vi "Generate Worker Types.vi"(11 "Worker lvlib":path) -> (0 "error out":errorcluster, 1 "Types":T1[](array[typedef]), 2 "Special Terminals":T5={"Action"=-1, "Init"=-1, "Tag"=-1, "State in"=-1, "State out"=-1, "Error"=-1, "Control"=-1}, 3 "Worker VI":refnum<vi>)   [LabVIEW 2022 SP3, in "FlexBlocks Support.lvlib"]
uses:
  FlexBlocks Support.lvlib
  Terminal Direction.ctl
  Value Mode.ctl
  Special Terminal.ctl
  Type Descriptor.ctl
  Special Terminal Indices.ctl
  <vilib>/Utility/Data Type/NI_Data Type.lvlib
  Worker Action.ctl
panel:
  out "Array":path[](array[path])
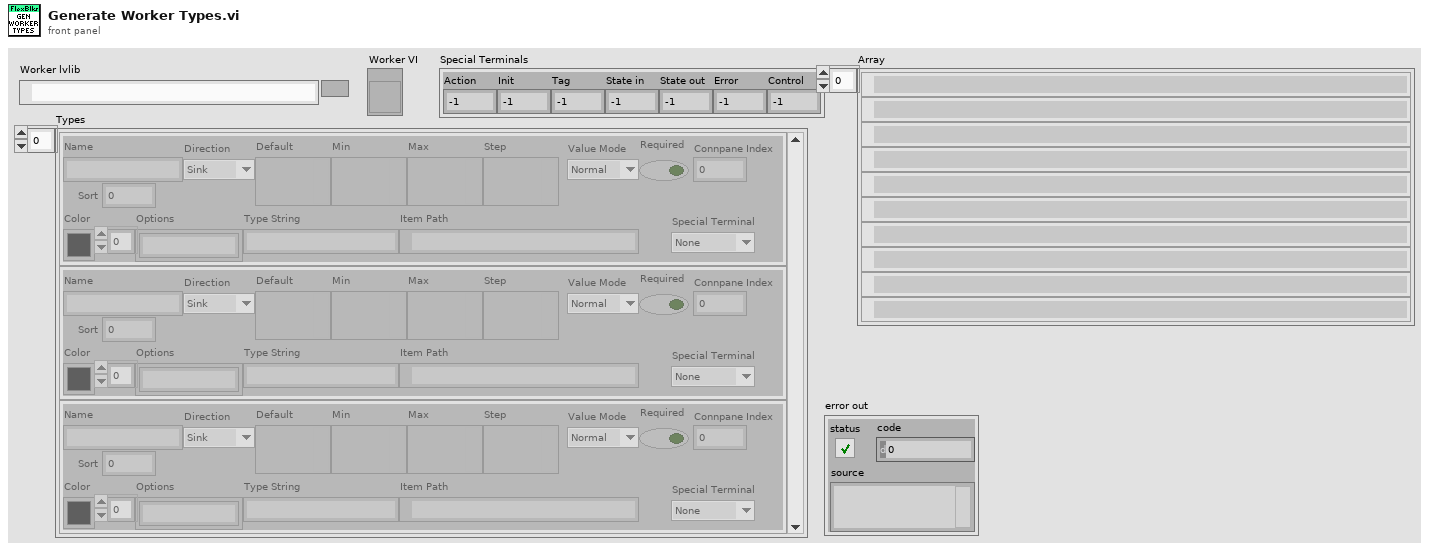
[diagram p1: front panel]
types:
  T1 = typedef "FlexBlocks Support.lvlib/Type Descriptor.ctl" = cluster{"Name":string, "Direction":T2, "Default":variant, "Min":variant, "Max":variant, "Step":variant, "Value Mode":T3, "Color":u32, "Options":string[], "Type String":string, "Item Path":path, "Required":bool, "Connpane Index":i32, "Special Terminal":T4, "Sort":i32}
  T2 = typedef "FlexBlocks Support.lvlib/Terminal Direction.ctl" = enum16{"Sink", "Source"}
  T3 = typedef "FlexBlocks Support.lvlib/Value Mode.ctl" = enum16{"Normal", "Range", "Select"}
  T4 = typedef "FlexBlocks Support.lvlib/Special Terminal.ctl" = enum16{"None", "Action", "Init", "Tag", "State in", "State out", "Error", "Control"}
  T5 = typedef "FlexBlocks Support.lvlib/Special Terminal Indices.ctl" = cluster{"Action":i32, "Init":i32, "Tag":i32, "State in":i32, "State out":i32, "Error":i32, "Control":i32}
  T6 = typedef "FlexBlocks Support.lvlib/Worker Action.ctl" = enum16{"Init", "Start", "Run", "Stop", "Close"}
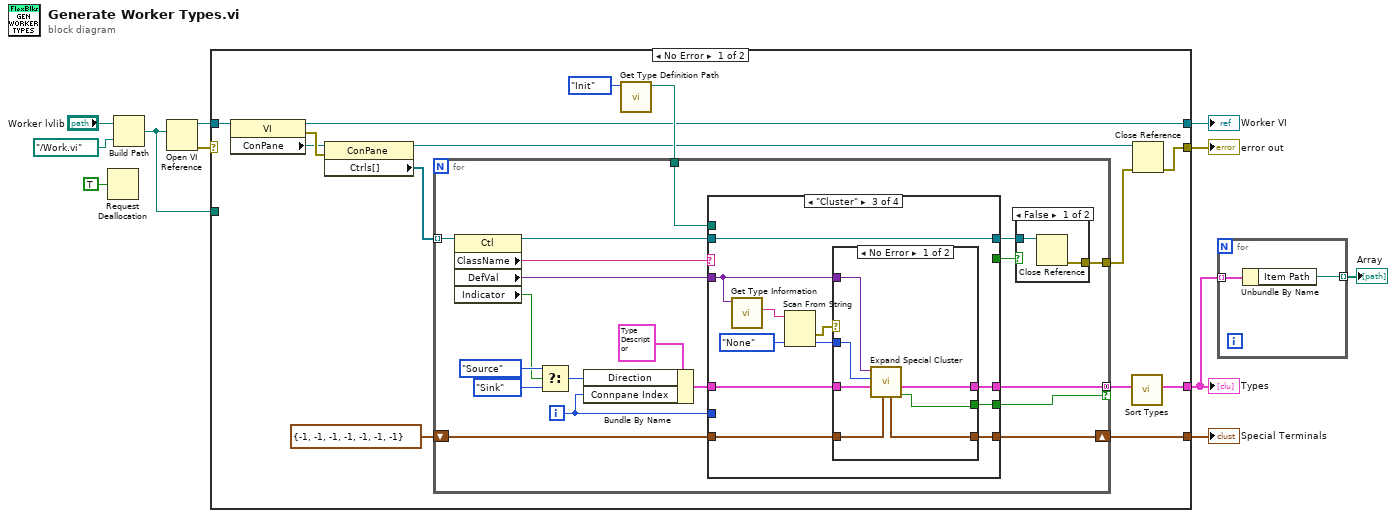
[diagram p0: block diagram]
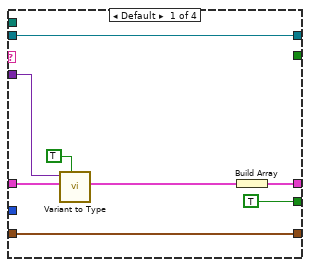
[diagram p3: hidden frame]
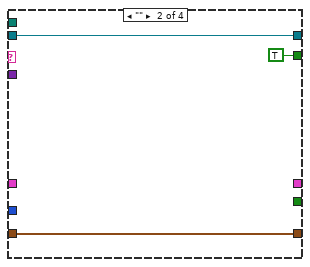
[diagram p4: hidden frame]
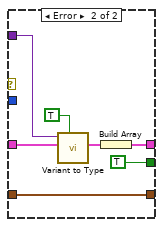
[diagram p5: hidden frame]
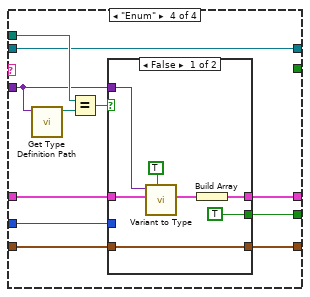
[diagram p6: hidden frame]
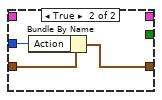
[diagram p7: hidden frame]
diagram:
  n1 = Request Deallocation(TRUE ("flag")) -> ()
  n2 = Build Path(base path="Worker lvlib", name or relative path=path "../Work.vi") -> (appended path=w6:path)
  n3 = Open VI Reference(vi path=w6) -> (vi reference=w8:refnum<vi>, error out=w7:errorcluster)  [unwired: 5 in]
  n4 = case shown="No Error" w7 {
    selector: w7 -> [_ w104]
    tunnel: w8 -> [w23 _]
    tunnel: w6 -> [_ _]
    tunnel: [w14 w104] -> w5
    tunnel: [w18 _] -> w4
    tunnel: [w15 _] -> w3
    tunnel: [w12 _] -> w2
    frame No Error {
      n5 = property class="VI"(reference=w23) -> (reference out=w15:refnum<vi>, error out=w25:errorcluster, "ConPane"=w24:refnum<vi>)  [unwired: 1 in]
      n6 = property class="ConPane"(reference=w24, error in=w25) -> (reference out=w16:refnum<vi>, "Ctrls[]"=w22:refnum<vi>[])  [unwired: 1 out]
      n7 = call <vilib>:"Get Type Definition Path.vi"("variant"=Worker_Action."Init" ("Worker Action")) -> ("type definition path"=w19:path)  [unwired: 9 in, 1 out]
      n8 = for {
        tunnel: w22 -> [w44] mode=indexing
        shift-right: [w32] -> w18
        shift-left: T5 {"Action"=-1, "Init"=-1, "Tag"=-1, "State in"=-1, "State out"=-1, "Error"=-1, "Control"=-1} ("Special Terminal Indices") -> [w38]
        tunnel: w19 -> [w34]
        tunnel: [w30] -> w17
        tunnel: [w29] -> w13 mode=concatenating if=w28
        i -> [w27]
        n9 = property class="Ctl"(reference=w44) -> (reference out=w33:refnum<vi>, "ClassName"=w36:string, "DefVal"=w35:variant, "Indicator"=w41:bool)  [unwired: 1 in, 1 out]
        n10 = Select(t=Terminal_Direction."Source" ("Direction"), s=w41, f=Terminal_Direction."Sink" ("Direction")) -> (s? t:f=w39:T2)
        n11 = Bundle By Name(cluster=T1 {"Name"="", "Direction"=enum."Sink", "Default"=variant, "Min"=variant, "Max"=variant, "Step"=variant, "Value Mode"=enum."Normal", "Color"=0, "Options"=[], "Type String"="", "Item Path"=path "", "Required"=FALSE, "Connpane Index"=0, "Special Terminal"=enum."None", "Sort"=0} ("Type Descriptor"), "Direction"=w39, "Connpane Index"=w27) -> (w37:T1)
        n12 = case shown="\"Cluster\"" w36 {
          tunnel: w38 -> [w53 w57 w61 w90]
          tunnel: w37 -> [w50 _ w62 w91]
          tunnel: w35 -> [w47 _ w63 w88]
          tunnel: w34 -> [_ _ _ w92]
          tunnel: w33 -> [w54 w56 w66 w87]
          tunnel: [w54 w56 w66 w87] -> w31
          tunnel: [w53 w57 w60 w85] -> w32
          tunnel: [w52 _ w59 w84] -> w29
          tunnel: [TRUE _ w58 w83] -> w28
          tunnel: w27 -> [_ _ _ w86]
          tunnel: [_ TRUE _ _] -> w26
          frame Default {
            n13 = call "Variant to Type.vi"("Required? (F)"=TRUE, "Type Descriptor in"=w50, "Variant"=w47) -> ("Type Descriptor"=w49:T1)  [unwired: 8 in]
            n14 = Build Array(w49) -> (w52:T1[])
          }
          frame "" {
          }
          frame "Cluster" {
            n15 = call <vilib>:"Get Type Information.vi"("variant"=w63) -> ("name"=w68:string)  [unwired: 6 in, 4 out]
            n16 = Scan From String(input string=w68, default 1=Special_Terminal."None" ("Special Terminal")) -> (error out=w65:errorcluster, output 1=w64:T4)  [unwired: 3 in, 2 out]
            n17 = case shown="No Error" w65 {
              tunnel: w64 -> [w72 _]
              tunnel: w63 -> [w71 w77]
              tunnel: w62 -> [w75 w81]
              tunnel: w61 -> [w73 w82]
              tunnel: [w70 w82] -> w60
              tunnel: [w74 w80] -> w59
              tunnel: [w69 TRUE] -> w58
              frame No Error {
                n18 = call "Expand Special Cluster.vi"("Special Terminal Indices in"=w73, "Type Descriptor"=w75, "Special Terminal"=w72, "Variant"=w71) -> ("Save Types?"=w69:bool, "Contained Types"=w74:T1[], "Special Terminal Indices"=w70:T5)  [unwired: 5 in]
              }
              frame Error {
                n19 = call "Variant to Type.vi"("Required? (F)"=TRUE, "Type Descriptor in"=w81, "Variant"=w77) -> ("Type Descriptor"=w78:T1)  [unwired: 8 in]
                n20 = Build Array(w78) -> (w80:T1[])
              }
            }
          }
          frame "Enum" {
            n21 = call <vilib>:"Get Type Definition Path.vi"("variant"=w88) -> ("type definition path"=w93:path)  [unwired: 9 in, 1 out]
            n22 = Equal?(x=w92, y=w93) -> (x = y?=w89:bool)
            n23 = case shown="False" w89 {
              tunnel: w91 -> [w99 _]
              tunnel: w90 -> [w100 w103]
              tunnel: w88 -> [w95 _]
              tunnel: w86 -> [_ w102]
              tunnel: [w100 w101] -> w85
              tunnel: [w97 _] -> w84
              tunnel: [TRUE _] -> w83
              frame False {
                n24 = call "Variant to Type.vi"("Required? (F)"=TRUE, "Type Descriptor in"=w99, "Variant"=w95) -> ("Type Descriptor"=w98:T1)  [unwired: 8 in]
                n25 = Build Array(w98) -> (w97:T1[])
              }
              frame True {
                n26 = Bundle By Name(cluster=w103, "Action"=w102) -> (w101:T5)
              }
            }
          }
        }
        n27 = case shown="False" w26 {
          tunnel: w31 -> [w46 _]
          tunnel: [w45 _] -> w30
          frame False {
            n28 = Close Reference(reference=w46) -> (error out=w45:errorcluster)  [unwired: 1 in]
          }
          frame True {
          }
        }
      }
      n29 = call "Sort Types.vi"("Types in"=w13) -> ("Types"=w12:T1[])  [unwired: 10 in]
      n30 = Close Reference(reference=w16, error in (no error)=w17) -> (error out=w14:errorcluster)
    }
    frame Error {
    }
  }
  "error out" <- w5
  "Special Terminals" <- w4
  "Worker VI" <- w3
  "Types" <- w2
  n31 = for {
    tunnel: w2 -> [w106] mode=indexing
    tunnel: [w105] -> w1 mode=indexing
    n32 = Unbundle By Name(w106) -> ("Item Path"=w105:path)
  }
  "Array" <- w1
